vi "Begin.vi"(8 "error in (no error)":errorcluster, 11 "Comp Elevator in":refnum<class "Comp Elevator.lvclass">) -> (0 "error out":errorcluster, 3 "Comp Elevator out":refnum<class "Comp Elevator.lvclass">)   [LabVIEW 2014, in "Comp Elevator.lvlib" / "Comp Elevator.lvclass"]
uses:
  Comp Elevator.lvclass
  Robot/Elevator/Elevator Class/Elevator.lvclass
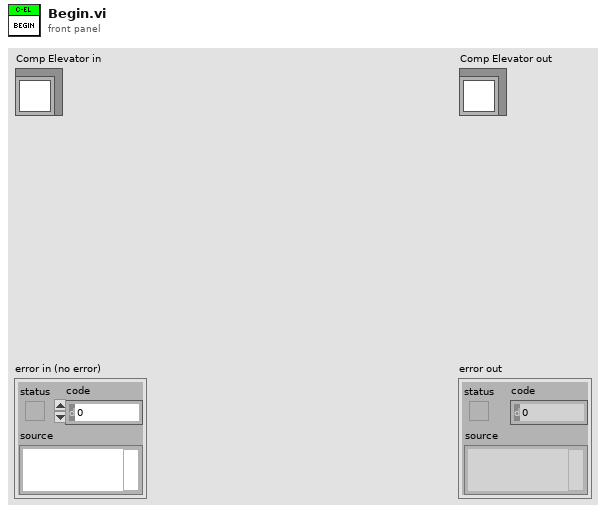
[diagram p1: front panel]
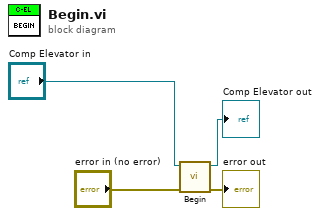
[diagram p0: block diagram]
diagram:
  n1 = call-parent "Begin.vi"("error in (no error)"="error in (no error)", "System Actor in"="Comp Elevator in") -> ("error out"=→"error out":errorcluster, "System Actor out"=→"Comp Elevator out":refnum<class "Comp Elevator.lvclass">)  [unwired: 8 in]
